vi "Update Error Status.vi"(8 "error in (no error)":errorcluster, 11 "navX Status in":refnum<class "navX Error Status.lvclass">) -> (0 "error out":errorcluster, 2 "Last Valid Timestamp (ms)":u32, 3 "navX Status out":refnum<class "navX Error Status.lvclass">)   [LabVIEW 2015, in "navX Library v3.lvlib" / "navX Error Status.lvclass"]
uses:
  navX Error Status.lvclass
  navX Error Status.lvclass/navX Error Status.ctl
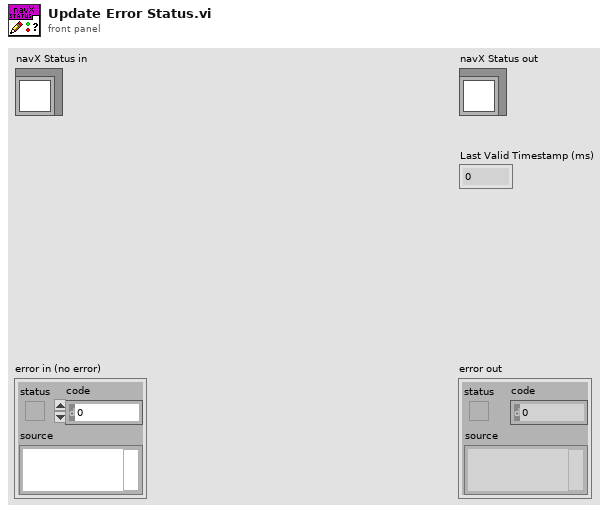
[diagram p1: front panel]
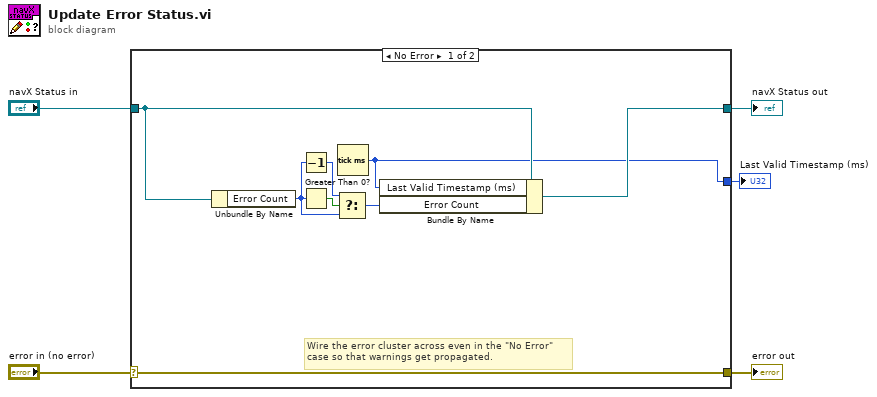
[diagram p0: block diagram]
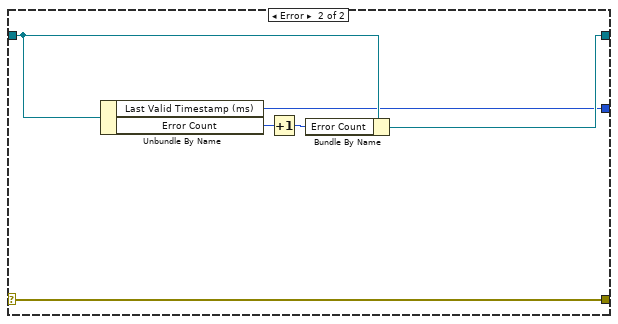
[diagram p2: hidden frame]
diagram:
  n1 = case shown="No Error" "error in (no error)" {
    selector: "error in (no error)" -> [w13 w19]
    tunnel: [w13 w19] -> w4
    tunnel: [w11 w15] -> w2
    tunnel: "navX Status in" -> [w12 w16]
    tunnel: [w6 w14] -> w1
    frame No Error {
      # "Wire the error cluster across even in the \"No Error\"\ncase so that warnings get propagated."
      n2 = Unbundle By Name(w12) -> ("Error Count"=w9:i32)
      n3 = Decrement(x=w9) -> (x-1=w8:i32)
      n4 = Greater Than 0?(x=w9) -> (x > 0?=w10:bool)
      n5 = Select(t=w8, s=w10, f=w9) -> (s? t:f=w7:i32)
      n6 = Tick Count (ms)() -> (millisecond timer value=w6:u32)
      n7 = Bundle By Name(cluster=w12, "Last Valid Timestamp (ms)"=w6, "Error Count"=w7) -> (w11:refnum<class "navX Error Status.lvclass">)
    }
    frame Error {
      n8 = Unbundle By Name(w16) -> ("Last Valid Timestamp (ms)"=w14:u32, "Error Count"=w18:i32)
      n9 = Increment(x=w18) -> (x+1=w17:i32)
      n10 = Bundle By Name(cluster=w16, "Error Count"=w17) -> (w15:refnum<class "navX Error Status.lvclass">)
    }
  }
  "error out" <- w4
  "navX Status out" <- w2
  "Last Valid Timestamp (ms)" <- w1
